vi "240126_Change_Z_Position.vi"(0 "Relative move (au)":u32=1, 5 "Z position":u32, 7 "-+ (FT)":bool, 11 "error in (no error)":errorcluster) -> (4 "Z position out":u32, 15 "error out":errorcluster)   [LabVIEW 2014]
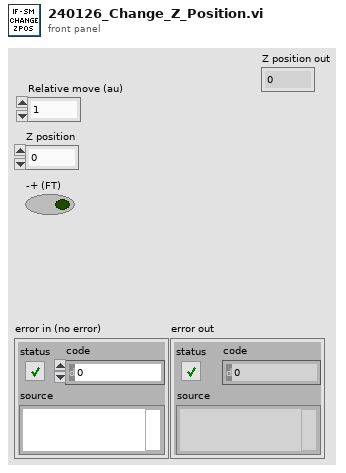
[diagram p1: front panel]
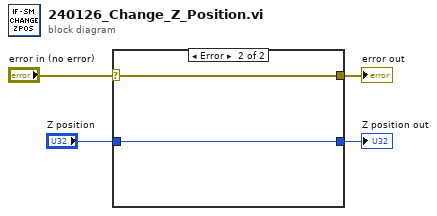
[diagram p0: block diagram]
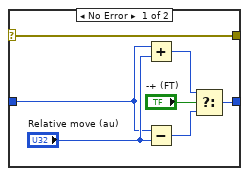
[diagram p2: hidden frame]
diagram:
  n1 = case shown="Error" "error in (no error)" {
    selector: "error in (no error)" -> [w11 w13]
    tunnel: [w11 w13] -> w3
    tunnel: "Z position" -> [w6 w12]
    tunnel: [w5 w12] -> w1
    frame No Error {
      n2 = Add(x=w6, y="Relative move (au)") -> (x+y=w7:u32)
      n3 = Subtract(x=w6, y="Relative move (au)") -> (x-y=w9:u32)
      n4 = Select(t=w7, s="-+ (FT)", f=w9) -> (s? t:f=w5:u32)
    }
    frame Error {
    }
  }
  "error out" <- w3
  "Z position out" <- w1
